vi "BL_SetHardConf.vi"(8 "error in (no error)":errorcluster, 9 "Hardware Configuration":T1 {"Instrument ground" items=["Grounded Mode", "Floating Mode"]; "Electrode connection" items=["Standard connection", "CE to ground connection", "WE to ground connection", "High Voltage Connection"]}, 10 "Channel":u8, 11 "Potentiostat Galvanostat in":refnum<class "Potentiostat Galvanostat.lvclass">) -> (0 "error out":errorcluster, 2 "Channel":u8, 3 "Potentiostat Galvanostat out":refnum<class "Potentiostat Galvanostat.lvclass">)   [LabVIEW 2018, in "Potentiostat Galvanostat.lvclass"]
doc: "The hardware conf object. The attribute “Conn” is the electrode\nconnection mode and the attribute “Ground” is the instrument\nground. See 5. Structures and Constants to have the value of these\nattributes."
uses:
  Potentiostat Galvanostat.lvclass
  Controls/Hardware Configuration.ctl
  Controls/Electrode Connection.ctl
  Controls/Electrode Mode.ctl
  Potentiostat Galvanostat.lvclass/Potentiostat Galvanostat.ctl
  BL_GetErrorMsg.vi
  <vilib>/Utility/error.llb/Error Cluster From Error Code.vi
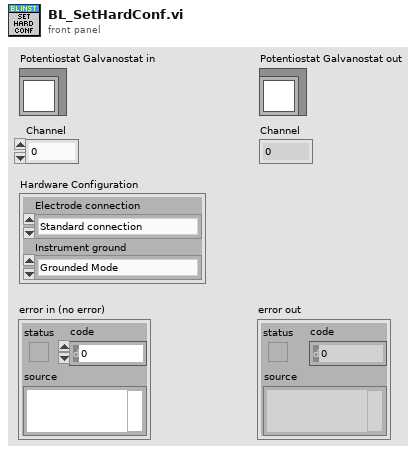
[diagram p1: front panel]
types:
  T1 = typedef "Potentiostat Galvanostat.lvclass/Hardware Configuration.ctl" = cluster{"Electrode connection":T2, "Instrument ground":T3}
  T2 = typedef "Potentiostat Galvanostat.lvclass/Electrode Connection.ctl" = i32
  T3 = typedef "Potentiostat Galvanostat.lvclass/Electrode Mode.ctl" = i32
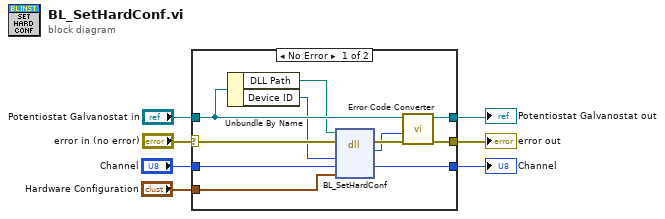
[diagram p0: block diagram]
diagram:
  n1 = case shown="No Error" "error in (no error)" {
    selector: "error in (no error)" -> [w15 w20]
    tunnel: [w18 w20] -> w6
    tunnel: [w17 w19] -> w4
    tunnel: "Potentiostat Galvanostat in" -> [w16 w19]
    tunnel: "Channel" -> [w14 _]
    tunnel: [w11 _] -> w2
    tunnel: "Hardware Configuration" -> [w8 _]
    frame No Error {
      n2 = Unbundle By Name(w16) -> ("DLL Path"=w12:path, "Device ID"=w13:i32)
      n3 = dll-call lib="C:/Program Files (x86)/National Instruments/LabVIEW 2018/user.lib/EClib/EClib.*" fn="BL_SetHardConf"(path in=w12, error in=w15, "Device ID"=w13, "Channel"=w14, w8) -> (error out=w10:errorcluster, "Error Code"=w9:i32, "Channel"=w11:u8)  [unwired: 3 in, 1 out]
      n4 = call "Error Code Converter.vi"("error in (no error)"=w10, "Error Code"=w9, "Potentiostat Galvanostat in"=w16) -> ("error out"=w18:errorcluster, "Potentiostat Galvanostat out"=w17:refnum<class "Potentiostat Galvanostat.lvclass">)  [unwired: 7 in]
    }
    frame Error {
    }
  }
  "error out" <- w6
  "Potentiostat Galvanostat out" <- w4
  "Channel" <- w2
